vi "UHR-Fleezers Control (host) -TL FB Corrected Ronen semipassive.vi"(0 "Tab Control":T5(tab)=enum."Trap Control (RF)") -> ()   [LabVIEW 2013] (continued)
                  n1350 = case shown="3" w2095 {
                    tunnel: [FALSE TRUE] -> w2096
                    frame 0, Default {
                    }
                    frame 3 {
                      n1351 = local write "Manipulating Trap"(FALSE ("Manipulating Trap")) -> ()
                    }
                  }
                }
              }
            }
          }
        }
      }
      event Mouse Move {
        n1352 = event-data() -> ()  [unwired: 6 out]
      }
    }
    n1353 = local read "Stop All"() -> (w1917:bool)
    n1354 = node-c288() -> ()  [unwired: 2 out]
  }
  n1355 = node-c288(w34) -> ()  [unwired: 1 out]
  n1356 = node-c288(w88) -> ()  [unwired: 1 out]
  n1357 = node-c288(w95) -> ()  [unwired: 1 out]
  n1358 = node-c288(i64 1 ("Period"), 1 ("Processor")) -> (w182:T25)  [unwired: 2 out]
  n1359 = timed-loop "Acquire Data" {
    tunnel: w44 -> [w2383]
    tunnel: w60 -> [w2382]
    tunnel: [w2413] -> w53
    tunnel: [w2407] -> w52
    timing: w182 -> [_]
    timing-out: [_] -> w181
    tunnel: w79 -> [w2219]
    stop <- "Stop All" stop-if-true
    (unwired) u32 0 ("Number of Elements")
    w2206 = "NI_ChannelName" ("name")
    n1360 = node-c288() -> ()  [unwired: 2 out]
    n1361 = First Call?() -> (First Call?: T/F=w2172:bool)
    n1362 = Or(x="Reset", y=w2172) -> (x .or. y?=w2173:bool)
    n1363 = local read "MCL Tracking"() -> (w2110:bool)
    n1364 = case "Reset data stream" shown="True" w2173 {
      tunnel: w2383 -> [w2525 w2533]
      tunnel: w2382 -> [w2524 w2532]
      tunnel: [w2525 w2527] -> w2108
      tunnel: [w2524 w2526] -> w2378
      frame False {
      }
      frame True {
        w2530 = TRUE ("AI to FIFO")
        n1365 = local write "Overflow (data lost)"(FALSE ("Overflow (data lost)")) -> ()
        n1366 = call "reset FPGA DMA.vi"("error in"=w2532, "FPGA VI Reference In"=w2533) -> ("error out"=w2528:errorcluster, "FPGA VI Reference Out"=w2529:T20)
        n1367 = xnode "Read/Write Control"("FPGA VI Reference In"=w2529, "error in"=w2528, "AI to FIFO"=w2530, "APD to FIFO"=w2530) -> ("FPGA VI Reference Out"=w2527:T20, "error out"=w2526:errorcluster)
      }
    }
    n1368 = Or(x="Start AOD Scan", y="Trap Raster Scan") -> (x .or. y?=w2334:bool)
    n1369 = case "Start AOM raster scan" shown="True" w2334 {
      tunnel: w2108 -> [w3262 w3272]
      tunnel: w2378 -> [w3261 w3271]
      tunnel: [w3262 w3265] -> w2107
      tunnel: [w3261 w3264] -> w2377
      frame False {
      }
      frame True {
        n1370 = case shown="True" "Restart DMA? (AOD)" {
          tunnel: [w3310 w3312] -> w3266
          tunnel: [w3309 w3311] -> w3267
          tunnel: w3272 -> [w3310 w3314]
          tunnel: w3271 -> [w3309 w3313]
          frame False {
          }
          frame True {
            n1371 = local write "Overflow (data lost)"(FALSE ("Overflow (data lost)")) -> ()
            n1372 = call "reset FPGA DMA.vi"("error in"=w3313, "FPGA VI Reference In"=w3314) -> ("error out"=w3311:errorcluster, "FPGA VI Reference Out"=w3312:T20)
          }
        }
        n1373 = local write "Trap Raster Scan"(FALSE ("Trap Raster Scan")) -> ()
        n1374 = case shown="True" "Move MCL Also?" {
          tunnel: w3267 -> [w3275 w3304]
          tunnel: w3266 -> [w3276 w3305]
          tunnel: [w3274 w3308] -> w3265
          tunnel: [w3273 w3307] -> w3264
          frame False {
            w3277 = TRUE ("AI to FIFO")
            n1375 = xnode "Read/Write Control"("FPGA VI Reference In"=w3276, "error in"=w3275, "AI to FIFO"=w3277, "APD to FIFO"=w3277, "Start scan"=w3277) -> ("FPGA VI Reference Out"=w3274:T20, "error out"=w3273:errorcluster)
          }
          frame True {
            w3301 = FALSE ("1D or 2D Scan?")
            w3306 = TRUE ("AI to FIFO")
            # "Count for MCL loop"
            # "N total cycles"
            # "N steps"
            # "V_int"
            n1376 = local read "Scan Range (nm)"() -> (w3283:dbl)
            n1377 = local read "Number of F/B Scans (AOD)"() -> (w3300:u16)
            n1378 = Sign(1:w3283) -> (0:w3282:dbl)
            n1379 = Compound Arithmetic op=MULTIPLY(w3283, "MCL Step Position Ratio", "MCL/AOM Scale Tweak") -> (w3287:dbl)
            n1380 = Negate(x=w3282) -> (-x=w3279:dbl)
            n1381 = Multiply(x=w3279, y="MCL Step Increment (V_int)") -> (x*y=w3281:dbl)
            n1382 = Divide(x=w3287, y="MCL X Cal (nm/V)") -> (x/y=w3293:dbl)
            n1383 = Multiply(x=32767.0 ("y"), y=w3293) -> (x*y=w3299:dbl)
            n1384 = local read "Total Counts (ticks)"() -> (w3284:u32)
            n1385 = local read "Cycles/step (AOD)"() -> (w3295:u64)
            n1386 = local read "Scan steps (AOD)"() -> (w3296:u64)
            n1387 = Divide(x=w3299, y=10.0) -> (x/y=w3292:dbl)
            n1388 = Divide(x=w3292, y="MCL Step Increment (V_int)") -> (x/y=w3290:dbl)
            n1389 = Absolute Value(x=w3290) -> (abs(x)=w3278:dbl)
            n1390 = Compound Arithmetic op=MULTIPLY(w3296, w3295, w3284) -> (w3291:u64)
            n1391 = local write "wait to reset values"(w3306) -> ()
            n1392 = local write "MCL Scanning"(w3306) -> ()
            n1393 = Divide(x=w3291, y=w3278) -> (x/y=w3288:dbl)
            "MCL Count" <- w3288
            n1394 = xnode "Read/Write Control"("FPGA VI Reference In"=w3305, "error in"=w3304, "Scan steps (MCL)"=w3278, "Number of scans (MCL)"=w3300, "Cycles per step (MCL)"=u64 1, "Scan freq.  increment (MCL)"=w3281, "1D or 2D Scan?"=w3301, "MCL Scan Axis"=w3301, "Cont. Scan (MCL)"=w3301, "MCL count"=w3288) -> ("FPGA VI Reference Out"=w3303:T20, "error out"=w3302:errorcluster)
            n1395 = xnode "Read/Write Control"("FPGA VI Reference In"=w3303, "error in"=w3302, "AI to FIFO"=w3306, "APD to FIFO"=w3306, "Start scan"=w3306, "Start scan (MCL)"=w3306) -> ("FPGA VI Reference Out"=w3308:T20, "error out"=w3307:errorcluster)
          }
        }
        "Raster Scanning..." <- TRUE ("Scanning...")
      }
    }
    n1396 = And(x="Save scans", y=w2334) -> (x .and. y?=w2376:bool)
    n1397 = Compound Arithmetic op=OR("Start MCL Scan", "Confocal Image", "Confocal Linescan") -> (w2332:bool)
    n1398 = And(x="Save Data (MCL)", y=w2332) -> (x .and. y?=w2375:bool)
    n1399 = case "Start MCL raster scan" shown="True" w2332 {
      tunnel: w2107 -> [w2816 w2831]
      tunnel: w2377 -> [w2815 w2830]
      tunnel: [w2816 w2826] -> w2142
      tunnel: [w2815 w2825] -> w2141
      tunnel: [FALSE w2824] -> w2361
      tunnel: "Start MCL Scan" -> [_ w2819]
      tunnel: "Confocal Image" -> [_ w2818]
      tunnel: "Confocal Linescan" -> [_ _]
      frame False {
      }
      frame True {
        w2824 = TRUE
        n1400 = case shown="True" "Restart DMA? (MCL)" {
          tunnel: [w2876 w2878] -> w2829
          tunnel: [w2875 w2877] -> w2828
          tunnel: w2831 -> [w2876 w2881]
          tunnel: w2830 -> [w2875 w2880]
          frame False {
          }
          frame True {
            n1401 = call "reset FPGA DMA.vi"("error in"=w2880, "FPGA VI Reference In"=w2881) -> ("error out"=w2877:errorcluster, "FPGA VI Reference Out"=w2878:T20)
            n1402 = local write "Overflow (data lost)"(FALSE ("Overflow (data lost)")) -> ()
          }
        }
        n1403 = case shown="False" w2819 {
          selector: w2819 -> [_ w2835]
          tunnel: w2818 -> [w2834 _]
          tunnel: [w2834 w2835] -> w2817
          frame False {
            n1404 = property on="2D or 1D Scan" class="Bool (strict)"("Val(Sgnl)"=w2834) -> ()  [unwired: 2 in, 2 out]
            n1405 = property on="Confocal Image" class="Bool (strict)"("Value"=FALSE ("Start Confocal Map")) -> ()  [unwired: 2 in, 2 out]
          }
          frame True {
          }
        }
        n1406 = local write "MCL Scanning"(w2824) -> ()
        n1407 = local read "AO1"() -> (w2821:dbl)
        n1408 = local read "AO2"() -> (w2820:dbl)
        n1409 = case shown="True" "Center Scan" {
          tunnel: w2829 -> [w2842 w2874]
          tunnel: w2828 -> [w2841 w2873]
          tunnel: [w2840 w2872] -> w2826
          tunnel: [w2839 w2871] -> w2825
          tunnel: [w2837 w2858] -> w2823
          tunnel: [w2836 w2857] -> w2822
          tunnel: w2821 -> [w2837 w2863]
          tunnel: w2820 -> [w2836 w2866]
          tunnel: w2817 -> [_ _]
          frame False {
            w2838 = TRUE ("AI to FIFO")
            n1410 = xnode "Read/Write Control"("FPGA VI Reference In"=w2842, "error in"=w2841, "AI to FIFO"=w2838, "APD to FIFO"=w2838, "Start scan (MCL)"=w2838) -> ("FPGA VI Reference Out"=w2840:T20, "error out"=w2839:errorcluster)
          }
          frame True {
            w2870 = TRUE ("AI to FIFO")
            n1411 = local read "Scan steps (MCL)"() -> (w2849:u64)
            n1412 = local read "Scan lines (y)"() -> (w2845:u64)
            n1413 = local read "Fast Scan Dir"() -> (w2856:bool)
            n1414 = local read "Actual MCL Inc (V)"() -> (w2846:dbl)
            n1415 = Decrement(x=w2845) -> (x-1=w2844:u64)
            n1416 = Decrement(x=w2849) -> (x-1=w2848:u64)
            n1417 = Multiply(x=w2846, y=w2844) -> (x*y=w2843:dbl)
            n1418 = Divide(x=w2843, y=2.0) -> (x/y=w2853:dbl)
            n1419 = Multiply(x=w2846, y=w2848) -> (x*y=w2847:dbl)
            n1420 = Divide(x=w2847, y=2.0) -> (x/y=w2852:dbl)
            n1421 = Select(t=w2852, s=w2856, f=w2853) -> (s? t:f=w2851:dbl)
            n1422 = Select(t=w2853, s=w2856, f=w2852) -> (s? t:f=w2855:dbl)
            n1423 = Subtract(x=w2863, y=w2855) -> (x-y=w2854:dbl)
            n1424 = Subtract(x=w2866, y=w2851) -> (x-y=w2850:dbl)
            n1425 = local read "2D or 1D Scan"() -> (w2868:bool)
            n1426 = Not(x=w2856) -> (.not. x?=w2862:bool)
            n1427 = Not(x=w2868) -> (.not. x?=w2864:bool)
            n1428 = And(x=w2856, y=w2864) -> (x .and. y?=w2865:bool)
            n1429 = And(x=w2864, y=w2862) -> (x .and. y?=w2867:bool)
            n1430 = Select(t=w2866, s=w2867, f=w2850) -> (s? t:f=w2857:dbl)
            n1431 = Select(t=w2863, s=w2865, f=w2854) -> (s? t:f=w2858:dbl)
            n1432 = call "Volt to I16.vi"("Voltage In"=w2858) -> ("I16 Voltage Out"=w2861:i16)
            n1433 = call "Volt to I16.vi"("Voltage In"=w2857) -> ("I16 Voltage Out"=w2860:i16)
            n1434 = xnode "Read/Write Control"("FPGA VI Reference In"=w2874, "error in"=w2873, "AI to FIFO"=w2870, "APD to FIFO"=w2870, "Start scan (MCL)"=w2870, "AO1"=w2861, "AO2"=w2860) -> ("FPGA VI Reference Out"=w2872:T20, "error out"=w2871:errorcluster)
          }
        }
        "Initial Y" <- w2823
        "Initial X" <- w2822
        "wait to reset values" <- w2824
      }
    }
    n1435 = local read "Trap Pos Elements/DMA read"() -> (w2215:u32)
    n1436 = local read "Trap AI Elements/DMA read"() -> (w2140:u32)
    n1437 = local read "APD Elements/DMA read"() -> (w2258:u32)
    n1438 = local read "Trap AI FIFO Depth"() -> (w2423:u32)
    n1439 = xnode "Invoke Method"("FPGA VI Reference In"=w2142, "error in"=w2141, "Number of Elements"=w2215, "Timeout (ms)"=-1) -> ("Data"=w2179:u16[], "Elements Remaining"=→"Trap Pos FIFO El Remaining":u32)  [unwired: 2 out]
    n1440 = xnode "Invoke Method"("FPGA VI Reference In"=w2142, "error in"=w2141, "Number of Elements"=w2140, "Timeout (ms)"=-1 ("Timeout")) -> ("FPGA VI Reference Out"=w2111:T20, "error out"=w2143:errorcluster, "Data"=w2139:i16[], "Elements Remaining"=w2144:u32)
    "Trap AI FIFO El. Rem." <- w2144
    n1441 = xnode "Get APD Data"("FPGA VI Reference In"=w2142, "error in"=w2141, "Number of Elements"=w2258, "Timeout (ms)"=-1) -> ("Data"=w2257:u32[], "Elements Remaining"=→"APD FIFO Elements Remaining":u32)  [unwired: 2 out]
    n1442 = Subtract(x=w2423, y=w2140) -> (x-y=w2422:u32)
    n1443 = Decimate 1D Array(w2179) -> (w2176:u16[], w2178:u16[], w2177:u16[])
    n1444 = Divide(x=w2144, y=w2422) -> (x/y=w2421:dbl)
    "Buffer Status" <- w2421
    n1445 = To Unsigned Long Integer(number=w2176) -> (unsigned 32bit integer=w2175:u32[])
    n1446 = Join Numbers(hi=w2178, lo=w2177) -> ((hi.lo)=w2174:u32[])
    n1447 = Equal?(x=w2421, y=1.0) -> (x = y?=w2419:bool)
    n1448 = Join Numbers(hi=w2175, lo=w2174) -> ((hi.lo)=w2168:u64[])
    n1449 = call "IR AOM word to freq - vec.vi"("Frequency Word In (double vec)"=w2168) -> ("Frequency Out"=w2214:dbl[])
    n1450 = case "Alert buffer overflow" shown="False" w2419 {
      frame False {
      }
      frame True {
        n1451 = call <vilib>:"Beep.vi"() -> ()  [unwired: 3 in, 9 out]
        "Overflow (data lost)" <- TRUE ("Overflow (data lost)")
      }
    }
    n1452 = Decimate 1D Array(w2214) -> (w2213:dbl[], w2212:dbl[])
    n1453 = Array Size(array=w2139) -> (size(s)=→"Waveform Chart":i32)
    n1454 = Build Array(w2213, w2212) -> (w2211:dbl[][])
    n1455 = local read "Trap Sets"() -> (w2294:u32)
    n1456 = case "Deinterlace trap data, average down PSD" shown="2" w2294 {
      tunnel: w2139 -> [w2911 w2976]
      tunnel: [w2908 w2973] -> w2287
      tunnel: [w2911 w2975] -> w2171
      tunnel: "Detector Type" -> [w2910 w2971]
      tunnel: [w2909 w2974] -> w2286
      tunnel: [w2907 w2972] -> w2394
      frame 1, Default {
        n1457 = Divide(x=w2911, y=3276.7) -> (x/y=w2912:dbl[])
        n1458 = Decimate 1D Array(w2912) -> (w2921:dbl[], w2920:dbl[], w2919:dbl[], w2918:dbl[], w2917:dbl[], w2916:dbl[], w2915:dbl[], w2914:dbl[])
        n1459 = case shown="\"IR-QPD + PSD + FB-QPD position\"" w2910 {
          tunnel: w2921 -> [w2945 w2970]
          tunnel: w2920 -> [w2944 w2969]
          tunnel: w2919 -> [w2929 w2947]
          tunnel: w2918 -> [w2930 w2957]
          tunnel: w2917 -> [w2943 w2968]
          tunnel: w2916 -> [w2942 w2967]
          tunnel: w2915 -> [w2926 w2948]
          tunnel: w2914 -> [w2925 w2946]
          tunnel: [w2924 w2954] -> w2909
          tunnel: [w2923 w2953] -> w2908
          tunnel: [w2922 w2952] -> w2907
          frame "IR-QPD + PSD + FB-QPD", Default {
            w2922 = 0  # Channel pattern
            n1460 = Divide(x=w2945, y=w2930) -> (x/y=w2932:dbl[])
            n1461 = Divide(x=w2944, y=w2930) -> (x/y=w2931:dbl[])
            n1462 = Divide(x=w2943, y=w2926) -> (x/y=w2928:dbl[])
            n1463 = Divide(x=w2942, y=w2925) -> (x/y=w2927:dbl[])
            n1464 = Build Array(w2932, w2931, w2930, w2929, w2928, w2927, w2926, w2925) -> (w2923:dbl[][])
            n1465 = Bundle("T1 Y", "T1 X", "T1 Sum", "FB Sum", "PSD Y", "PSD X", "PSD Y Sum", "PSD X Sum") -> (w2941:T42)  [unwired: 1 out]
            n1466 = Cluster To Array(cluster=w2941) -> (array=w2924:string[])
          }
          frame "IR-QPD + PSD + FB-QPD position" {
            w2952 = 3  # Channel pattern
            n1467 = Negate(x=w2948) -> (-x=w2949:dbl[])
            n1468 = Divide(x=w2970, y=w2957) -> (x/y=w2959:dbl[])
            n1469 = Divide(x=w2969, y=w2957) -> (x/y=w2958:dbl[])
            n1470 = Divide(x=w2968, y=w2948) -> (x/y=w2956:dbl[])
            n1471 = Divide(x=w2967, y=w2949) -> (x/y=w2955:dbl[])
            n1472 = Build Array(w2959, w2958, w2957, w2946, w2947, w2956, w2955, w2948) -> (w2953:dbl[][])
            n1473 = Bundle("T1 Y", "T1 X", "T1 Sum", "FB X", "FB Sum", "PSD Y", "PSD X", "PSD Y Sum") -> (w2966:T42)  [unwired: 1 out]
            n1474 = Cluster To Array(cluster=w2966) -> (array=w2954:string[])
          }
        }
      }
      frame 2 {
        n1475 = case shown="\"UCB Fleezers 052511\"" w2971 {
          tunnel: w2976 -> [w3038 w3105 w3133 w3240]
          tunnel: [w2977 w3097 w3128 w3171] -> w2975
          tunnel: [w3004 w3088 w3130 w3218] -> w2974
          tunnel: [w3003 w3052 w3107 w3185] -> w2973
          tunnel: [w2997 w3087 w3170 w3216] -> w2972
          frame "IR-QPD + PSD + FB-QPD", Default {
            w2997 = 1  # Channel pattern
            # "time average x2 the 4th signal and the 4 psd signals (detection laser)"
            # "deinterlace 3 signals from qpd"
            n1476 = Decimate 1D Array(w3038) -> (w3037:i16[], w3036:i16[], w3002:i16[], w3035:i16[], w3025:i16[], w3023:i16[], w3022:i16[], w3020:i16[])
            n1477 = call "downsample 1D array - double.vi"("Ave N"=2.0, "Array In"=w3025) -> ("Array Out"=w3024:dbl[])  [unwired: 1 out]
            n1478 = call "downsample 1D array - double.vi"("Ave N"=2.0, "Array In"=w3020) -> ("Array Out"=w3019:dbl[])  [unwired: 1 out]
            n1479 = call "downsample 1D array - double.vi"("Ave N"=2.0, "Array In"=w3022) -> ("Array Out"=w3021:dbl[])  [unwired: 1 out]
            n1480 = call "downsample 1D array - double.vi"("Ave N"=2.0, "Array In"=w3023) -> ("Array Out"=w3005:dbl[])  [unwired: 1 out]
            n1481 = Decimate 1D Array(w3037) -> (w3034:i16[], w3006:i16[])
            n1482 = Decimate 1D Array(w3036) -> (w3033:i16[], w3031:i16[])
            n1483 = Decimate 1D Array(w3035) -> (w3032:i16[], w3030:i16[])
            n1484 = Decimate 1D Array(w3002) -> (w3001:i16[], w3000:i16[])
            n1485 = Interleave 1D Arrays(w3034, w3033, w3032, w3006, w3031, w3030, w3001, w3000, w3024, w3005, w3021, w3019) -> (w3018:dbl[])
            n1486 = To Word Integer(number=w3018) -> (16bit integer=w2977:i16[])
            n1487 = Divide(x=w3018, y=3276.7) -> (x/y=w3017:dbl[])
            n1488 = Decimate 1D Array(w3017) -> (w3016:dbl[], w3015:dbl[], w3014:dbl[], w3013:dbl[], w3012:dbl[], w3011:dbl[], w2999:dbl[], w2998:dbl[], w3010:dbl[], w3009:dbl[], w3008:dbl[], w3007:dbl[])
            n1489 = Divide(x=w3016, y=w3014) -> (x/y=w2984:dbl[])
            n1490 = Divide(x=w3015, y=w3014) -> (x/y=w2983:dbl[])
            n1491 = Divide(x=w3013, y=w3011) -> (x/y=w2982:dbl[])
            n1492 = Divide(x=w3012, y=w3011) -> (x/y=w2981:dbl[])
            n1493 = Divide(x=w3010, y=w3008) -> (x/y=w2980:dbl[])
            n1494 = Divide(x=w3009, y=w3007) -> (x/y=w2979:dbl[])
            n1495 = Bundle("T1 Y", "T1 X", "T1 Sum", "T2 Y", "T2 X", "T2 Sum", "T1 FB Sum", "T2 FB Sum", "PSD Y", "PSD X", "PSD Y Sum", "PSD X Sum") -> (w2985:T43)  [unwired: 1 out]
            n1496 = Build Array(w2984, w2983, w3014, w2982, w2981, w3011, w2999, w2998, w2980, w2979, w3008, w3007) -> (w3003:dbl[][])
            n1497 = Cluster To Array(cluster=w2985) -> (array=w3004:string[])
          }
          frame "IR-QPD + PSD + FB-QPD X position" {
            w3087 = 2  # Channel pattern
            # "convert\nADC numbers\nto volts"
            # "time average x2 the 3 psd signals (detection laser)"
            # "deinterlace 3 signals from qpds"
            n1498 = Decimate 1D Array(w3105) -> (w3104:i16[], w3103:i16[], w3040:i16[], w3041:i16[], w3050:i16[], w3047:i16[], w3044:i16[], w3075:i16[])
            n1499 = Decimate 1D Array(w3104) -> (w3102:i16[], w3089:i16[])
            n1500 = call "downsample 1D array - I16.vi"("Ave N"=2.0, "Array In"=w3050) -> ("Array Out"=w3048:i16[])  [unwired: 1 in]
            n1501 = call "downsample 1D array - I16.vi"("Ave N"=2.0, "Array In"=w3047) -> ("Array Out"=w3045:i16[])  [unwired: 1 in]
            n1502 = Decimate 1D Array(w3103) -> (w3101:i16[], w3099:i16[])
            n1503 = Decimate 1D Array(w3041) -> (w3100:i16[], w3098:i16[])
            n1504 = Decimate 1D Array(w3075) -> (w3074:i16[], w3072:i16[])
            n1505 = Decimate 1D Array(w3040) -> (w3073:i16[], w3071:i16[])
            n1506 = call "downsample 1D array - I16.vi"("Ave N"=2.0, "Array In"=w3044) -> ("Array Out"=w3042:i16[])  [unwired: 1 in]
            n1507 = Interleave 1D Arrays(w3102, w3101, w3100, w3089, w3099, w3098, w3074, w3073, w3072, w3071, w3048, w3045, w3042) -> (w3097:i16[])
            n1508 = Divide(x=w3097, y=3276.7) -> (x/y=w3096:dbl[])
            n1509 = Decimate 1D Array(w3096) -> (w3095:dbl[], w3094:dbl[], w3093:dbl[], w3092:dbl[], w3091:dbl[], w3090:dbl[], w3063:dbl[], w3061:dbl[], w3060:dbl[], w3058:dbl[], w3057:dbl[], w3056:dbl[], w3053:dbl[])
            n1510 = Divide(x=w3095, y=w3093) -> (x/y=w3079:dbl[])
            n1511 = Divide(x=w3094, y=w3093) -> (x/y=w3078:dbl[])
            n1512 = Divide(x=w3092, y=w3090) -> (x/y=w3077:dbl[])
            n1513 = Divide(x=w3091, y=w3090) -> (x/y=w3076:dbl[])
            n1514 = Divide(x=w3063, y=w3061) -> (x/y=w3062:dbl[])
            n1515 = Divide(x=w3060, y=w3058) -> (x/y=w3059:dbl[])
            n1516 = Divide(x=w3057, y=w3053) -> (x/y=w3055:dbl[])
            n1517 = Negate(x=w3053) -> (-x=w3051:dbl[])
            n1518 = Divide(x=w3056, y=w3051) -> (x/y=w3054:dbl[])
            n1519 = Bundle("T1 Y", "T1 X", "T1 Sum", "T2 Y", "T2 X", "T2 Sum", "T1 FB X", "T1 FB Sum", "T2 FB X", "T2 FB Sum", "PSD Y", "PSD X", "PSD Y Sum") -> (w3080:T44)  [unwired: 1 out]
            n1520 = Build Array(w3079, w3078, w3093, w3077, w3076, w3090, w3062, w3061, w3059, w3058, w3055, w3054, w3053) -> (w3052:dbl[][])
            n1521 = Cluster To Array(cluster=w3080) -> (array=w3088:string[])
          }
          frame "UCB Fleezers 052511" {
            w3170 = 2  # Channel pattern
            n1522 = Decimate 1D Array(w3133) -> (w3168:i16[], w3167:i16[], w3132:i16[], w3131:i16[], w3125:i16[], w3122:i16[], w3121:i16[], w3120:i16[])
            n1523 = Decimate 1D Array(w3168) -> (w3166:i16[], w3151:i16[])
            n1524 = Decimate 1D Array(w3167) -> (w3165:i16[], w3163:i16[])
            n1525 = Decimate 1D Array(w3132) -> (w3164:i16[], w3162:i16[])
            n1526 = Decimate 1D Array(w3131) -> (w3127:i16[], w3126:i16[])
            n1527 = Decimate 1D Array(w3125) -> (w3124:i16[], w3123:i16[])
            n1528 = call "downsample 1D array - I16.vi"("Ave N"=2.0, "Array In"=w3122) -> ("Array Out"=w3119:i16[])  [unwired: 1 in]
            n1529 = call "downsample 1D array - I16.vi"("Ave N"=2.0, "Array In"=w3121) -> ("Array Out"=w3118:i16[])  [unwired: 1 in]
            n1530 = call "downsample 1D array - I16.vi"("Ave N"=2.0, "Array In"=w3120) -> ("Array Out"=w3117:i16[])  [unwired: 1 in]
            n1531 = Interleave 1D Arrays(w3166, w3165, w3164, w3151, w3163, w3162, w3127, w3124, w3126, w3123, w3119, w3118, w3117) -> (w3128:i16[])
            n1532 = Divide(x=w3128, y=3276.7) -> (x/y=w3158:dbl[])
            n1533 = Decimate 1D Array(w3158) -> (w3157:dbl[], w3156:dbl[], w3155:dbl[], w3154:dbl[], w3153:dbl[], w3152:dbl[], w3116:dbl[], w3114:dbl[], w3113:dbl[], w3111:dbl[], w3110:dbl[], w3109:dbl[], w3108:dbl[])
            n1534 = Divide(x=w3157, y=w3155) -> (x/y=w3138:dbl[])
            n1535 = Divide(x=w3156, y=w3155) -> (x/y=w3137:dbl[])
            n1536 = Divide(x=w3154, y=w3152) -> (x/y=w3136:dbl[])
            n1537 = Divide(x=w3153, y=w3152) -> (x/y=w3135:dbl[])
            n1538 = Divide(x=w3116, y=w3114) -> (x/y=w3115:dbl[])
            n1539 = Divide(x=w3113, y=w3111) -> (x/y=w3112:dbl[])
            n1540 = Bundle("T1 Y", "T1 X", "T1 Sum", "T2 Y", "T2 X", "T2 Sum", "T1 FB X", "T2 FB Sum", "T2 FB X", "T2 FB Sum", "PSD Y", "PSD X", "PSD Sum") -> (w3139:T44)  [unwired: 1 out]
            n1541 = Build Array(w3138, w3137, w3155, w3136, w3135, w3152, w3115, w3114, w3112, w3111, w3110, w3109, w3108) -> (w3107:dbl[][])
            n1542 = Cluster To Array(cluster=w3139) -> (array=w3130:string[])
          }
          frame "IR-QPD + PSD + FB-QPD XY positions" {
            w3216 = 4  # Channel pattern
            # "time average x2 the 3 psd signals (detection laser)"
            # "deinterlace 3 signals from qpds"
            n1543 = Decimate 1D Array(w3240) -> (w3239:i16[], w3238:i16[], w3217:i16[], w3237:i16[], w3183:i16[], w3229:i16[], w3228:i16[], w3205:i16[])
            n1544 = Decimate 1D Array "QPD Y"(w3239) -> (w3236:i16[], w3219:i16[])
            n1545 = call "downsample 1D array - double.vi"("Ave N"=2.0, "Array In"=w3229) -> ("Array Out"=w3204:dbl[])  [unwired: 1 out]
            n1546 = call "downsample 1D array - double.vi"("Ave N"=2.0, "Array In"=w3228) -> ("Array Out"=w3203:dbl[])  [unwired: 1 out]
            n1547 = Decimate 1D Array "Feedback Sum"(w3217) -> (w3201:i16[], w3199:i16[])
            n1548 = Decimate 1D Array "Feedback Y"(w3183) -> (w3182:i16[], w3181:i16[])
            n1549 = Decimate 1D Array "Feedback X"(w3205) -> (w3202:i16[], w3200:i16[])
            n1550 = Decimate 1D Array "QPD Sum"(w3237) -> (w3234:i16[], w3232:i16[])
            n1551 = Decimate 1D Array "QPD X"(w3238) -> (w3235:i16[], w3233:i16[])
            n1552 = Interleave 1D Arrays(w3236, w3235, w3234, w3219, w3233, w3232, w3182, w3202, w3201, w3181, w3200, w3199, w3204, w3203) -> (w3227:dbl[])
            n1553 = To Word Integer(number=w3227) -> (16bit integer=w3171:i16[])
            n1554 = Divide(x=w3227, y=3276.7) -> (x/y=w3226:dbl[])
            n1555 = Decimate 1D Array(w3226) -> (w3225:dbl[], w3224:dbl[], w3223:dbl[], w3222:dbl[], w3221:dbl[], w3220:dbl[], w3178:dbl[], w3192:dbl[], w3176:dbl[], w3177:dbl[], w3190:dbl[], w3174:dbl[], w3188:dbl[], w3186:dbl[])
            n1556 = Divide(x=w3225, y=w3223) -> (x/y=w3209:dbl[])
            n1557 = Divide(x=w3224, y=w3223) -> (x/y=w3208:dbl[])
            n1558 = Divide(x=w3222, y=w3220) -> (x/y=w3207:dbl[])
            n1559 = Divide(x=w3221, y=w3220) -> (x/y=w3206:dbl[])
            n1560 = Divide(x=w3178, y=w3176) -> (x/y=w3175:dbl[])
            n1561 = Divide(x=w3192, y=w3176) -> (x/y=w3191:dbl[])
            n1562 = Divide(x=w3177, y=w3174) -> (x/y=w3173:dbl[])
            n1563 = Divide(x=w3190, y=w3174) -> (x/y=w3189:dbl[])
            n1564 = Negate(x=w3186) -> (-x=w3184:dbl[])
            n1565 = Divide(x=w3188, y=w3184) -> (x/y=w3187:dbl[])
            n1566 = Bundle("T1 Y", "T1 X", "T1 Sum", "T2 Y", "T2 X", "T2 Sum", "T1 FB Y", "T1 FB X", "T1 FB Sum", "T2 FB Y", "T2 FB X", "T2 FB Sum", "PSD X", "PSD Y Sum") -> (w3172:T45)  [unwired: 1 out]
            n1567 = Build Array(w3209, w3208, w3223, w3207, w3206, w3220, w3175, w3191, w3176, w3173, w3189, w3174, w3187, w3186) -> (w3185:dbl[][])
            n1568 = Cluster To Array(cluster=w3172) -> (array=w3218:string[])
          }
        }
      }
    }
    "AI labels" <- w2286
    n1569 = xnode "Read/Write Control"("FPGA VI Reference In"=w2111) -> ("FPGA VI Reference Out"=w2104:T20, "BD1 Frequency Out 1"=w2125:u64)  [unwired: 1 in, 1 out]
    n1570 = local read "BD 1 Frequency 2 (MHz)"() -> (w2116:dbl)
    n1571 = To Double Precision Float(number=w2125) -> (double precision float=w2122:dbl)
    n1572 = Multiply(x=49125000.0, y=6.0) -> (x*y=w2121:dbl)
    n1573 = Multiply(x=w2122, y=w2121) -> (x*y=w2119:dbl)
    n1574 = Scale By Power Of 2(n=-48, x=w2119) -> (x*2^n=w2118:dbl)
    n1575 = local read "Dynamic Force FB"() -> (w2115:bool)
    n1576 = local read "Trap Pos. FB ON"() -> (w2114:bool)
    n1577 = Divide(x=w2118, y=1000000.0) -> (x/y=w2109:dbl)
    n1578 = case shown="True" w2110 {
      tunnel: w2109 -> [_ w2500]
      tunnel: w2107 -> [_ w2487]
      frame False {
      }
      frame True {
        n1579 = local read "AOM X Cal (nm/MHz)"() -> (w2497:dbl)
        n1580 = local read "Zero T1 position"() -> (w2499:dbl)
        n1581 = Subtract(x=w2500, y=w2499) -> (x-y=w2498:dbl)
        n1582 = Multiply(x=w2498, y=w2497) -> (x*y=w2496:dbl)
        n1583 = local read "MCL X Cal (nm/V)"() -> (w2493:dbl)
        n1584 = Multiply(x=w2496, y="Tracking factor") -> (x*y=w2494:dbl)
        n1585 = local read "Zero MCL x position"() -> (w2492:dbl)
        n1586 = Divide(x=w2494, y=w2493) -> (x/y=w2491:dbl)
        n1587 = Add(x=w2492, y=w2491) -> (x+y=w2484:dbl)
        "Current MCL (V)" <- w2484
        n1588 = Multiply(x=w2484, y=32767.0) -> (x*y=w2488:dbl)
        n1589 = Divide(x=w2488, y=10.0) -> (x/y=w2485:dbl)
        n1590 = To Word Integer(number=w2485) -> (16bit integer=w2486:i16)
        n1591 = xnode "Read/Write Control"("FPGA VI Reference In"=w2487, "AO2"=w2486) -> ()  [unwired: 1 in, 2 out]
      }
    }
    n1592 = Subtract(x=w2116, y=w2109) -> (x-y=w2105:dbl)
    "Current deltaFreq" <- w2105
    n1593 = Compound Arithmetic op=AND(w2115, w2114, "Real time offset \ncorrection for setpoint") -> (w2112:bool)
    n1594 = case shown="True" w2112 {
      tunnel: w2105 -> [_ w2503]
      tunnel: w2104 -> [_ w2502]
      frame False {
      }
      frame True {
        n1595 = local read "T1 kappa_x (pN/nm)"() -> (w2511:dbl)
        n1596 = local read "T1 alpha_x (nm/V)"() -> (w2512:dbl)
        n1597 = local read "Negate offset difference"() -> (w2513:bool)
        n1598 = local read "Offset file step size"() -> (w2521:dbl)
        n1599 = Multiply(x="Target Force (pN)", y=2.0) -> (x*y=w2509:dbl)
        n1600 = local read "Setpoint offset\nCorrection values"() -> (w2518:dbl[])
        n1601 = Divide(x=w2503, y=w2521) -> (x/y=w2520:dbl)
        n1602 = Select(t=-1, s=w2513, f=1) -> (s? t:f=w2514:i32)
        n1603 = To Long Integer(number=w2520) -> (32bit integer=w2519:i32)
        n1604 = Multiply(x=w2512, y=w2511) -> (x*y=w2508:dbl)
        n1605 = Divide(x=w2509, y=w2508) -> (x/y=w2507:dbl)
        n1606 = Index Array(array=w2518, index=w2519) -> (element=w2517:dbl)
        n1607 = Multiply(x=w2514, y=w2517) -> (x*y=w2506:dbl)
        n1608 = Add(x=w2507, y=w2506) -> (x+y=w2505:dbl)
        n1609 = To Fixed-Point(number=w2505) -> (fixed-point=w2501:fxp<+/-,16,1>)  [unwired: 1 in]
        "Actual setpoint" <- w2501
        n1610 = xnode "Read/Write Control"("FPGA VI Reference In"=w2502, "Trap Pos. FB SP"=w2501) -> ()  [unwired: 1 in, 2 out]
      }
    }
    n1611 = case shown="False" "Take full offset data for display" {
      tunnel: [w2470 w2476] -> w2311
      tunnel: [w2469 w2475] -> w2309
      tunnel: w2105 -> [_ w2482]
      frame False {
        n1612 = Divide(x="T2 offset_x (mV)", y=1000.0) -> (x/y=w2469:dbl)
        n1613 = Divide(x="T1 offset_x (mV)", y=1000.0) -> (x/y=w2470:dbl)
      }
      frame True {
        n1614 = local read "Offset Values"() -> (w2483:T14)
        n1615 = local read "Offset file step size"() -> (w2481:dbl)
        n1616 = Unbundle By Name(w2483) -> ("Trap 1X offset"=w2478:dbl[], "Trap 2X offset"=w2477:dbl[])
        n1617 = Divide(x=w2482, y=w2481) -> (x/y=w2480:dbl)
        n1618 = To Long Integer(number=w2480) -> (32bit integer=w2479:i32)
        n1619 = Index Array(array=w2478, index=w2479) -> (element=w2476:dbl)
        n1620 = Index Array(array=w2477, index=w2479) -> (element=w2475:dbl)
      }
    }
    n1621 = Decimate 1D Array(w2257) -> (w2284:u32[], w2221:u32[])
    n1622 = local read "DMA Update Period (s)"() -> (w2295:dbl)
    n1623 = local read "BD 1 Frequency 2 (MHz)"() -> (w2163:dbl)
    n1624 = local read "BD 1 Frequency 1 (MHz)"() -> (w2164:dbl)
    n1625 = Build Array(w2284, w2221) -> (w2358:u32[][])
    n1626 = local read "Data Period (s)"() -> (w2270:dbl)
    n1627 = Decimate 1D Array(w2171) -> (w2194:i16[], w2193:i16[], w2191:i16[], w2190:i16[])  [unwired: 9 out]
    n1628 = To Double Precision Float(number=w2358) -> (double precision float=w2359:dbl[][])
    n1629 = local read "APD Integration Time (s)"() -> (w2234:dbl)
    n1630 = Divide(x=w2194, y=w2193) -> (x/y=w2195:dbl[])
    n1631 = Divide(x=w2191, y=w2190) -> (x/y=w2192:dbl[])
    n1632 = feedback #1(0.0) -> (w2208:dbl)
    n1633 = Add(x=w2295, y=w2208) -> (x+y=w2396:dbl)
    n1634 = feedback-in #1(w2396) -> ()
    n1635 = local read "AOM X Cal (nm/MHz)"() -> (w2161:dbl)
    n1636 = To Time Stamp(1:w2208) -> (0:w2207:timestamp)
    n1637 = Split 1D Array(array=w2195, index="N El. to Ave.") -> (second subarray=w2198:dbl[])  [unwired: 1 out]
    n1638 = Split 1D Array(array=w2192, index="N El. to Ave.") -> (second subarray=w2197:dbl[])  [unwired: 1 out]
    n1639 = local read "Trap X AI1 (DMA)"() -> (w2196:T13)
    n1640 = Multiply(x=w2270, y="Trap Disp. Downsample") -> (x*y=w2209:dbl)
    "Display Period (s)" <- w2209
    n1641 = Bundle("BD 1 Frequency 1 (MHz)"=w2164, "BD 1 Frequency 2 (MHz)"=w2163) -> (w2165:T46)  [unwired: 1 out]
    n1642 = for "Trap AI" {
      tunnel: [w2906] -> w2390 mode=indexing
      tunnel: w2207 -> [w2896]
      tunnel: "Trap Disp. Downsample" -> [w2904]
      tunnel: w2287 -> [w2902] mode=indexing
      tunnel: w2270 -> [w2901]
      tunnel: w2286 -> [w2900] mode=indexing
      tunnel: w2206 -> [w2899]
      tunnel: [w2898] -> w2245 mode=indexing
      tunnel: w2209 -> [w2897]
      n1643 = Bundle By Name("Y"=w2902, "dt"=w2901) -> (w2903:waveform(dbl))  [unwired: 1 out]
      n1644 = Set Waveform Attribute(5:w2900, 6:w2899, 7:w2903) -> (3:w2898:waveform(dbl))  [unwired: 1 in, 2 out]
      n1645 = call "downsample 1D array - double.vi"("Ave N"=w2904, "Array In"=w2902) -> ("Array Out"=w2905:dbl[])  [unwired: 1 out]
      n1646 = Bundle By Name(cluster=w2898, "t0"=w2896, "Y"=w2905, "dt"=w2897) -> (w2906:waveform(dbl))
    }
    n1647 = call-poly <vilib>:"Mean.vi"("X"=w2197) -> ("mean"=w2185:dbl)  [unwired: 1 out]
    n1648 = call-poly <vilib>:"Mean.vi"("X"=w2198) -> ("mean"=w2186:dbl)  [unwired: 1 out]
    n1649 = Cluster To Array(cluster=w2165) -> (array=w2162:dbl[])
    n1650 = Reciprocal(x=w2209) -> (1/x=→"Trap Disp. Freq. (Hz)":dbl)
    n1651 = local read "Data points/scans (MCL)"() -> (w2370:dbl)
    n1652 = To Fixed-Point(number=w2185) -> (fixed-point=w2183:fxp<+/-,16,1>)  [unwired: 1 in]
    n1653 = To Fixed-Point(number=w2186) -> (fixed-point=w2184:fxp<+/-,16,1>)  [unwired: 1 in]
    n1654 = Bundle("Trap 1 Pos.", "Trap 2 Pos.") -> (w2205:cluster{string, string})  [unwired: 1 out]
    n1655 = Bundle By Name(cluster=w2196, "Set 1"=w2184, "Set 2"=w2183) -> (→"Trap X AI1 (DMA)":T13)
    n1656 = Cluster To Array(cluster=w2205) -> (array=w2202:string[])
    n1657 = for "Trap Position" {
      tunnel: w2211 -> [w2546] mode=indexing
      tunnel: "Trap Disp. Downsample" -> [w2545]
      tunnel: w2209 -> [w2543]
      tunnel: w2207 -> [w2542]
      tunnel: w2206 -> [w2540]
      tunnel: w2202 -> [w2539] mode=indexing
      tunnel: [w2538] -> w2160 mode=indexing
      tunnel: w2162 -> [w2536] mode=indexing
      tunnel: w2161 -> [w2534]
      n1658 = call "downsample 1D array - double.vi"("Ave N"=w2545, "Array In"=w2546) -> ("Array Out"=w2544:dbl[])  [unwired: 1 out]
      n1659 = Subtract(x=w2544, y=w2536) -> (x-y=w2537:dbl[])
      n1660 = Multiply(x=w2534, y=w2537) -> (x*y=w2535:dbl[])
      n1661 = Bundle By Name("Y"=w2535, "dt"=w2543, "t0"=w2542) -> (w2541:waveform(dbl))  [unwired: 1 out]
      n1662 = Set Waveform Attribute(5:w2539, 6:w2540, 7:w2541) -> (3:w2538:waveform(dbl))  [unwired: 1 in, 2 out]
    }
    "Trap Positions" <- w2160
    n1663 = Bundle("APD 1", "APD 2") -> (w2389:cluster{string, string})  [unwired: 1 out]
    n1664 = Cluster To Array(cluster=w2389) -> (array=w2386:string[])
    n1665 = for "APD" {
      tunnel: w2359 -> [w2885] mode=indexing
      tunnel: w2234 -> [w2893]
      tunnel: [w2889] -> w2241 mode=indexing
      tunnel: "APD Disp. Scale" -> [w2890]
      tunnel: w2206 -> [w2888]
      tunnel: w2386 -> [w2887] mode=indexing
      tunnel: "APD Disp. Downsample" -> [w2883]
      tunnel: [w2886] -> w2385
      tunnel: w2207 -> [w2882]
      n1666 = call "integrate 1D array interval - double.vi"("Ave N"=w2883, "Array In"=w2885) -> ("Array Out"=w2884:dbl[])  [unwired: 1 out]
      n1667 = Multiply(x=w2893, y=w2883) -> (x*y=w2886:dbl)
      n1668 = Divide(x=w2884, y=w2890) -> (x/y=w2891:dbl[])
      n1669 = Bundle By Name("t0"=w2882, "Y"=w2891, "dt"=w2886) -> (w2892:waveform(dbl))  [unwired: 1 out]
      n1670 = Set Waveform Attribute(5:w2887, 6:w2888, 7:w2892) -> (3:w2889:waveform(dbl))  [unwired: 1 in, 2 out]
    }
    "APD Display Period (s)" <- w2385
    n1671 = Reciprocal(x=w2385) -> (1/x=→"APD Display Freq. (Hz)":dbl)
    n1672 = local read "Display Period (s)"() -> (w2269:dbl)
    n1673 = Increment(x=w2370) -> (x+1=w2371:dbl)
    n1674 = Index Array(array=w2160, index=0) -> (element=w2158:waveform(dbl))
    n1675 = To Double Precision Float(number=w2284) -> (double precision float=w2283:dbl[])
    n1676 = feedback #2(w2371) -> (w2374:dbl)
    n1677 = Select(t=0, s=w2361, f=w2374) -> (s? t:f=w2367:dbl)
    n1678 = Array Size(array=w2283) -> (size(s)=w2373:i32)
    n1679 = Add(x=w2373, y=w2367) -> (x+y=w2368:dbl)
    n1680 = Unbundle By Name(w2158) -> ("Y"=w2156:dbl[])
    n1681 = feedback #3(w2284) -> (w2357:u32[])
    n1682 = Build Array (concatenate)(w2357, w2284) -> (w2354:u32[])
    n1683 = feedback #4(w2221) -> (w2240:u32[])
    n1684 = Divide(x="Bead Sep. Int. Time (s)", y=w2269) -> (x/y=w2154:dbl)
    n1685 = Build Array (concatenate)(w2240, w2221) -> (w2239:u32[])
    n1686 = Greater?(x=w2368, y=w2370) -> (0:w2369:bool)
    n1687 = feedback #5(w2156) -> (w2157:dbl[])
    n1688 = Build Array (concatenate)(w2156, w2157) -> (w2155:dbl[])
    n1689 = Select(t=w2367, s=w2369, f=w2368) -> (s? t:f=w2366:dbl)
    n1690 = feedback-in #2(w2366) -> ()
    n1691 = Array Size(array=w2354) -> (size(s)=w2351:i32)
    n1692 = Array Size(array=w2284) -> (size(s)=w2353:i32)
    n1693 = local read "MCL Scanning"() -> (w2364:bool)
    n1694 = local read "APD Integration Time (s)"() -> (w2248:dbl)
    n1695 = Build Array (concatenate)(w2241, w2390) -> (w2243:waveform(dbl)[])
    "All Signals" <- w2243
    n1696 = Split 1D Array(array=w2155, index=w2154) -> (first subarray=w2148:dbl[])  [unwired: 1 out]
    n1697 = feedback-in #5(w2148) -> ()
    n1698 = Multiply(x=w2353, y="APD Ave N") -> (x*y=w2352:dbl)
    n1699 = Greater?(x=w2351, y=w2352) -> (0:w2355:bool)
    n1700 = Not(x=w2369) -> (.not. x?=w2363:bool)
    n1701 = To Double Precision Float(number=w2221) -> (double precision float=w2220:dbl[])
    n1702 = call-poly <vilib>:"Mean.vi"("X"=w2148) -> ("mean"=w2147:dbl)  [unwired: 1 out]
    "Mean T1 Position (nm)" <- w2147
    n1703 = Subtract(x=w2148, y=w2147) -> (x-y=w2153:dbl[])
    n1704 = Square(x=w2153) -> (x^2=w2152:dbl[])
    n1705 = And(x=w2363, y=w2364) -> (x .and. y?=w2365:bool)
    n1706 = call-poly <vilib>:"Mean.vi"("X"=w2152) -> ("mean"=w2151:dbl)  [unwired: 1 out]
    n1707 = case shown="True" w2355 {
      tunnel: w2354 -> [w2666 w2673]
      tunnel: [w2666 w2671] -> w2300
      tunnel: w2352 -> [_ w2668]
      tunnel: w2351 -> [_ w2672]
      tunnel: w2239 -> [w2665 w2670]
      tunnel: [w2665 w2667] -> w2236
      frame False {
      }
      frame True {
        n1708 = Subtract(x=w2672, y=w2668) -> (x-y=w2669:dbl)
        n1709 = Array Subset(array=w2673, index=w2669, length=w2668) -> (w2671:u32[])
        n1710 = Array Subset(array=w2670, index=w2669, length=w2668) -> (w2667:u32[])
      }
    }
    n1711 = feedback-in #3(w2300) -> ()
    n1712 = feedback-in #4(w2236) -> ()
    n1713 = Or(x=w2365, y=w2361) -> (x .or. y?=w2362:bool)
    n1714 = Square Root(x=w2151) -> (sqrt(x)=w2150:dbl)
    n1715 = Equal?(x="Tab Control 6", y=T36."High Res Display") -> (x = y?=w2290:bool)
    n1716 = Multiply(x="APD Disp. Scale", y=w2241) -> (x*y=w2250:waveform(dbl)[])
    n1717 = Multiply(x="APD Disp. Downsample", y=w2248) -> (x*y=w2246:dbl)
    n1718 = Multiply(x=10.0, y=w2150) -> (x*y=→"Trap 1 Position RMS (A)":dbl)
    n1719 = Divide(x=w2250, y=w2246) -> (x/y=w2218:waveform(dbl)[])
    n1720 = Index Array(array=w2218, index=0) -> (element=w2228:waveform(dbl))
    n1721 = case "For computing FFTs for display" shown="True" "Compute FFT" {
      tunnel: w2245 -> [_ w3343]
      frame False {
      }
      frame True {
        n1722 = Build Array("FFT 1 Choice 1", "FFT 1 Choice 2", "FFT 2 Choice 1", "FFT 2 Choice 2") -> (w3336:u16[])
        n1723 = Array Size(array=w3343) -> (size(s)=w3342:i32)
        n1724 = feedback-in #6(w3336) -> ()
        n1725 = feedback #6(u16[] [100, 100, 100, 100]) -> (w3337:u16[])
        n1726 = feedback-in #7("# Spectra to Ave.") -> ()
        n1727 = feedback #7("# Spectra to Ave.") -> (w3334:dbl)
        n1728 = Not Equal?(x="# Spectra to Ave.", y=w3334) -> (x != y?=w3333:bool)
        n1729 = Not Equal?(x=w3336, y=w3337) -> (x != y?=w3335:bool)
        n1730 = feedback #8(1.0) -> (w3320:dbl)
        n1731 = Compound Arithmetic op=OR("Reset FFT", w3335, w3333) -> (w3318:bool)
        n1732 = Select(t=1.0, s=w3318, f=w3320) -> (s? t:f=w3322:dbl)
        n1733 = Greater?(x=w3322, y="# Spectra to Ave.") -> (0:w3341:bool)
        n1734 = Increment(x=w3322) -> (x+1=w3321:dbl)
        n1735 = feedback-in #8(w3321) -> ()
        n1736 = local read "DMA Update Period (s)"() -> (w3316:dbl)
        n1737 = Multiply(x="# Spectra to Ave.", y=w3316) -> (x*y=→"Ave. Time (s)":dbl)
        n1738 = Build Array(cluster{"f0":dbl, "df":dbl, "magnitude":dbl[]} {"f0"=0.0, "df"=0.0, "magnitude"=[]} ("PSD")) -> (w3325:cluster{"f0":dbl, "df":dbl, "magnitude":dbl[]}[])
        n1739 = Build Array(w3325, w3325, w3325, w3325) -> (w3327:T47)
        n1740 = feedback #9(w3327) -> (w3332:T47)
        n1741 = for {
          N: 4 -> [_]
          tunnel: w3336 -> [w3365] mode=indexing
          tunnel: w3343 -> [w3366]
          tunnel: w3342 -> [w3368]
          tunnel: w3318 -> [w3361]
          tunnel: w3341 -> [w3360]
          tunnel: "# Spectra to Ave." -> [w3359]
          tunnel: [w3358] -> w3331 mode=indexing
          tunnel: w3332 -> [w3363] mode=indexing
          tunnel: [w3362] -> w3319 mode=indexing
          tunnel: w3322 -> [w3357]
          n1742 = Less?(x=w3365, y=w3368) -> (x < y?=w3367:bool)
          n1743 = Index Array(array=w3366, index=w3365) -> (element=w3364:waveform(dbl))
          n1744 = case shown="True" w3367 {
            tunnel: w3364 -> [_ w3385]
            tunnel: w3363 -> [w3370 w3383]
            tunnel: [w3370 w3371] -> w3362
            tunnel: w3361 -> [_ w3382]
            tunnel: w3360 -> [_ w3375]
            tunnel: w3359 -> [_ w3374]
            tunnel: [cluster{"f0":dbl, "df":dbl, "magnitude":dbl[]} {"f0"=0.0, "df"=0.0, "magnitude"=[]} ("PSD") w3376] -> w3358
            tunnel: w3357 -> [_ w3373]
            frame False {
            }
            frame True {
              n1745 = call <vilib>:"Std Deviation and Variance.vi"("X"=w3385) -> ("mean"=w3386:dbl)  [unwired: 1 in, 2 out]
              n1746 = Subtract(x=w3385, y=w3386) -> (x-y=w3384:waveform(dbl))
              n1747 = xnode "Spectral Measurements"("Signals"=w3384) -> ("PSD"=w3378:cluster{"f0":dbl, "df":dbl, "magnitude":dbl[]})  [unwired: 1 in, 1 out]
              n1748 = case shown="False" w3382 {
                tunnel: w3383 -> [w3395 _]
                tunnel: [w3391 w3400] -> w3371
                tunnel: w3378 -> [w3394 w3401]
                tunnel: w3375 -> [w3393 _]
                frame False {
                  n1749 = Build Array (concatenate)(w3395, w3394) -> (w3392:cluster{"f0":dbl, "df":dbl, "magnitude":dbl[]}[])
                  n1750 = case shown="True" w3393 {
                    tunnel: w3392 -> [w3396 w3399]
                    tunnel: [w3396 w3397] -> w3391
                    frame False {
                    }
                    frame True {
                      n1751 = Delete From Array(array=w3399, index=0) -> (array with subset deleted=w3397:cluster{"f0":dbl, "df":dbl, "magnitude":dbl[]}[])  [unwired: 1 in, 1 out]
                    }
                  }
                }
                frame True {
                  n1752 = Build Array(w3401) -> (w3400:cluster{"f0":dbl, "df":dbl, "magnitude":dbl[]}[])
                }
              }
              n1753 = for {
                tunnel: w3371 -> [w3390] mode=indexing
                tunnel: [w3389] -> w3381 mode=indexing
                workers-P: _ -> [_]
                n1754 = Unbundle By Name(w3390) -> ("magnitude"=w3389:dbl[])
              }
              n1755 = Transpose 2D Array(2D array=w3381) -> (transposed array=w3380:dbl[][])
              n1756 = for {
                tunnel: w3380 -> [w3388] mode=indexing
                tunnel: [w3387] -> w3379 mode=indexing
                workers-P: _ -> [_]
                n1757 = Add Array Elements(numeric array=w3388) -> (sum=w3387:dbl)
              }
              n1758 = Select(t=w3374, s=w3375, f=w3373) -> (s? t:f=w3372:dbl)
              n1759 = Divide(x=w3379, y=w3372) -> (x/y=w3377:dbl[])
              n1760 = Bundle By Name(cluster=w3378, "magnitude"=w3377) -> (w3376:cluster{"f0":dbl, "df":dbl, "magnitude":dbl[]})
            }
          }
        }
        n1761 = case shown="True" w3318 {
          tunnel: w3319 -> [w3350 w3356]
          tunnel: [w3350 w3351] -> w3317
          frame False {
          }
          frame True {
            n1762 = Array Subset(array=w3356, index (row)=0 ("index"), length (row)=4 ("length"), index (col)=0 ("index"), length (col)=1 ("length")) -> (w3351:T47)
          }
        }
        n1763 = feedback-in #9(w3317) -> ()
        n1764 = Split 1D Array(array=w3331, index=2) -> (first subarray=→"FFT 1":cluster{"f0":dbl, "df":dbl, "magnitude":dbl[]}[], second subarray=→"FFT 2":cluster{"f0":dbl, "df":dbl, "magnitude":dbl[]}[])
      }
    }
    n1765 = Index Array(array=w2218, index=1) -> (element=w2226:waveform(dbl))
    n1766 = case "For displaying the high resolution display (no downsampling)" shown="True" w2290 {
      tunnel: w2245 -> [_ w2566]
      frame False {
      }
      frame True {
        n1767 = Index Array(array=w2566, index="High Res. Display") -> (element=w2567:waveform(dbl))
        n1768 = call <vilib>:"Std Deviation and Variance.vi"("X"=w2567) -> ("mean"=w2574:dbl, "standard deviation"=w2579:dbl)  [unwired: 1 in, 1 out]
        "Mean Intensity" <- w2574
        "Sigma" <- w2579
        n1769 = Subtract(x=w2567, y=w2574) -> (x-y=w2573:waveform(dbl))
        n1770 = Select(t=w2573, s="Subtract mean", f=w2567) -> (s? t:f=→"1 Channel":waveform(dbl))
        n1771 = Divide(x=w2579, y=w2574) -> (x/y=→"Sigma/Mean":dbl)
        n1772 = feedback #10(1) -> (w2568:i32)
        n1773 = Greater Or Equal?(x=w2568, y="Slow mean N ave.") -> (x >= y?=w2581:bool)
        n1774 = Increment(x=w2568) -> (x+1=w2583:i32)
        n1775 = Select(t=1, s=w2581, f=w2583) -> (s? t:f=w2570:i32)
        n1776 = feedback-in #10(w2570) -> ()
        n1777 = feedback #11() -> (w2571:waveform(dbl))  [unwired: 1 out]
        n1778 = case shown="Default" w2568 {
          tunnel: [w2586 w2589] -> w2572
          tunnel: w2571 -> [w2588 _]
          tunnel: w2567 -> [w2587 w2589]
          frame Default {
            n1779 = call-poly <vilib>:"Append Waveforms.vi"("waveform B"=w2587, "waveform A"=w2588) -> ("waveform out"=w2586:waveform(dbl))  [unwired: 1 in, 8 out]
          }
          frame 1 {
          }
        }
        n1780 = feedback-in #11(w2572) -> ()
        n1781 = case shown="True" w2581 {
          tunnel: w2572 -> [_ w2585]
          frame False {
          }
          frame True {
            n1782 = call-poly <vilib>:"Mean.vi"("X"=w2585) -> ("mean"=→"Slow mean":dbl)  [unwired: 1 out]
          }
        }
      }
    }
    n1783 = case "For plotting results of scanning MCL" shown="True" w2362 {
      tunnel: w2361 -> [_ w2706]
      tunnel: w2283 -> [_ w2802]
      tunnel: w2370 -> [_ _]
      tunnel: w2245 -> [_ w2776]
      tunnel: w2220 -> [_ w2707]
      tunnel: w2219 -> [_ w2680]
      frame False {
      }
      frame True {
        w2687 = u32 0 items=["Horizontal", "Vertical", "Central", "1st Diagonal", "2nd Diagonal"] ("Type of Symmetry")
        w2715 = u32 0 items=["Horizontal", "Vertical", "Central", "1st Diagonal", "2nd Diagonal"] ("Type of Symmetry")
        w2718 = u32 0 items=["Horizontal", "Vertical", "Central", "1st Diagonal", "2nd Diagonal"] ("Type of Symmetry")
        w2747 = u32 0 items=["Horizontal", "Vertical", "Central", "1st Diagonal", "2nd Diagonal"] ("Type of Symmetry")
        n1784 = Index Array(array=w2776, index=10) -> (element=w2782:waveform(dbl))
        n1785 = Index Array(array=w2776, index=11) -> (element=w2779:waveform(dbl))
        n1786 = local read "Cycles/step (MCL)"() -> (w2732:u64)
        n1787 = Index Array(array=w2776, index="Channel") -> (element=w2778:waveform(dbl))
        n1788 = Unbundle(w2680) -> ("New Image"=w2679:T3, "New Image"=w2678:T3, "New Image"=w2677:T3, "New Image"=w2676:T3)
        n1789 = Unbundle By Name(w2782) -> ("Y"=w2734:dbl[])
        n1790 = Unbundle By Name(w2779) -> ("Y"=w2736:dbl[])
        n1791 = Unbundle By Name(w2778) -> ("Y"=w2741:dbl[])
        n1792 = call "downsample 1D array - double.vi"("Ave N"=w2732, "Array In"=w2734) -> ("Array Out"=w2733:dbl[])  [unwired: 1 out]
        n1793 = call "downsample 1D array - double.vi"("Ave N"=w2732, "Array In"=w2736) -> ("Array Out"=w2735:dbl[])  [unwired: 1 out]
        n1794 = call "downsample 1D array - double.vi"("Ave N"=w2732, "Array In"=w2741) -> ("Array Out"=w2740:dbl[])  [unwired: 1 out]
        n1795 = feedback #12(w2802) -> (w2803:dbl[])
        n1796 = Build Array (concatenate)(w2803, w2802) -> (w2784:dbl[])
        n1797 = feedback #13(w2707) -> (w2709:dbl[])
        n1798 = Build Array (concatenate)(w2709, w2707) -> (w2708:dbl[])
        n1799 = local read "Scan steps (MCL)"() -> (w2689:u64)
        n1800 = Select(t=w2802, s=w2706, f=w2784) -> (s? t:f=w2788:dbl[])
        n1801 = feedback-in #12(w2788) -> ()
        n1802 = Select(t=w2707, s=w2706, f=w2708) -> (s? t:f=w2690:dbl[])
        n1803 = feedback-in #13(w2690) -> ()
        n1804 = local read "Scan lines (y)"() -> (w2675:u64)
        n1805 = local read "N APD Samp/step"() -> (w2691:dbl)
        n1806 = feedback #14(w2733) -> (w2790:dbl[])
        n1807 = Build Array (concatenate)(w2790, w2733) -> (w2781:dbl[])
        n1808 = feedback #15(w2740) -> (w2800:dbl[])
        n1809 = Build Array (concatenate)(w2800, w2740) -> (w2799:dbl[])
        n1810 = feedback #16(w2735) -> (w2792:dbl[])
        n1811 = Build Array (concatenate)(w2792, w2735) -> (w2793:dbl[])
        n1812 = Select(t=w2733, s=w2706, f=w2781) -> (s? t:f=w2737:dbl[])
        n1813 = feedback-in #14(w2737) -> ()
        n1814 = Select(t=w2740, s=w2706, f=w2799) -> (s? t:f=w2739:dbl[])
        n1815 = feedback-in #15(w2739) -> ()
        n1816 = Select(t=w2735, s=w2706, f=w2793) -> (s? t:f=w2738:dbl[])
        n1817 = feedback-in #16(w2738) -> ()
        n1818 = Multiply(x=w2689, y=u64 2) -> (x*y=w2674:u64)
        n1819 = call "integrate 1D array interval - double.vi"("Ave N"=w2691, "Array In"=w2690) -> ("Array Out"=w2702:dbl[])  [unwired: 1 out]
        n1820 = call "integrate 1D array interval - double.vi"("Ave N"=w2691, "Array In"=w2788) -> ("Array Out"=w2787:dbl[])  [unwired: 1 out]
        n1821 = Array Size(array=w2702) -> (size(s)=w2703:i32)
        n1822 = Array Size(array=w2787) -> (size(s)=w2789:i32)
        n1823 = Multiply(x=w2675, y=w2674) -> (x*y=w2705:u64)
        n1824 = Multiply(x=w2675, y=w2674) -> (x*y=w2797:u64)
        n1825 = call-poly <vilib>:"Mean.vi"("X"=w2737) -> ("mean"=w2721:dbl)  [unwired: 1 out]
        n1826 = Subtract(x=w2705, y=w2703) -> (x-y=w2696:u64)
        n1827 = call-poly <vilib>:"Mean.vi"("X"=w2739) -> ("mean"=w2726:dbl)  [unwired: 1 out]
        n1828 = call-poly <vilib>:"Mean.vi"("X"=w2738) -> ("mean"=w2724:dbl)  [unwired: 1 out]
        n1829 = call-poly <vilib>:"Mean.vi"("X"=w2702) -> ("mean"=w2693:dbl)  [unwired: 1 out]
        n1830 = Subtract(x=w2797, y=w2789) -> (x-y=w2731:u64)
        n1831 = call-poly <vilib>:"Mean.vi"("X"=w2787) -> ("mean"=w2728:dbl)  [unwired: 1 out]
        n1832 = Initialize Array(1.0 ("element"), w2696) -> (w2692:dbl[])
        n1833 = Initialize Array(1.0 ("element"), w2731) -> (w2722:dbl[])
        n1834 = Multiply(x=w2692, y=w2693) -> (x*y=w2694:dbl[])
        n1835 = Multiply(x=w2722, y=w2724) -> (x*y=w2725:dbl[])
        n1836 = Multiply(x=w2722, y=w2726) -> (x*y=w2727:dbl[])
        n1837 = Multiply(x=w2722, y=w2721) -> (x*y=w2723:dbl[])
        n1838 = Multiply(x=w2722, y=w2728) -> (x*y=w2729:dbl[])
        n1839 = Build Array (concatenate)(w2737, w2723) -> (w2791:dbl[])
        n1840 = Build Array (concatenate)(w2739, w2727) -> (w2795:dbl[])
        n1841 = Build Array (concatenate)(w2738, w2725) -> (w2794:dbl[])
        n1842 = Build Array (concatenate)(w2702, w2694) -> (w2704:dbl[])
        n1843 = Build Array (concatenate)(w2787, w2729) -> (w2796:dbl[])
        n1844 = Reshape Array(w2791, w2675, w2674) -> (w2757:dbl[][])
        n1845 = Reshape Array(w2704, w2675, w2674) -> (w2700:dbl[][])
        n1846 = Reshape Array(w2795, w2675, w2674) -> (w2749:dbl[][])
        n1847 = Reshape Array(w2794, w2675, w2674) -> (w2764:dbl[][])
        n1848 = Reshape Array(w2796, w2675, w2674) -> (w2774:dbl[][])
        n1849 = Array Subset(array=w2764, index (col)=0 ("index"), length (col)=w2689) -> (w2769:dbl[][])  [unwired: 2 in]
        n1850 = Array Subset(array=w2764, index (col)=w2689) -> (w2767:dbl[][])  [unwired: 3 in]
        n1851 = Array Subset(array=w2749, index (col)=0 ("index"), length (col)=w2689) -> (w2755:dbl[][])  [unwired: 2 in]
        n1852 = Array Subset(array=w2749, index (col)=w2689) -> (w2753:dbl[][])  [unwired: 3 in]
        n1853 = Array Subset(array=w2700, index (col)=0 ("index"), length (col)=w2689) -> (w2699:dbl[][])  [unwired: 2 in]
